vi "ActionVIOnCompile.vi"(8 "error in (no error)":errorcluster, 11 "Device Item Ref in":T1 format="%.0x") -> (0 "error out":errorcluster)   [LabVIEW 2020, in "gRPC Data Server System Explorer.lvlib"]
uses:
  gRPC Data Server System Explorer.lvlib
  <vilib>/NI VeriStand/Custom Device API/Custom Device Item Ref.ctl
  Shared/Compiled.Settings.ctl
  <vilib>/NI VeriStand/Custom Device Tools/Custom Device Utility Library/NI VeriStand - Search for Item by Name.vi
  <vilib>/NI VeriStand/Custom Device API/Set Item Property (Variant).vi
  <vilib>/NI VeriStand/Custom Device Tools/Custom Device Utility Library/Custom Device Utility Library.lvlib
  <vilib>/NI VeriStand/Custom Device API/Custom Device API.lvlib
  <vilib>/NI/NIVS Inline Async API/_Data Access System Explorer/Data Access System Explorer.lvlib
  Shared/gRPC Data Server Shared.lvlib
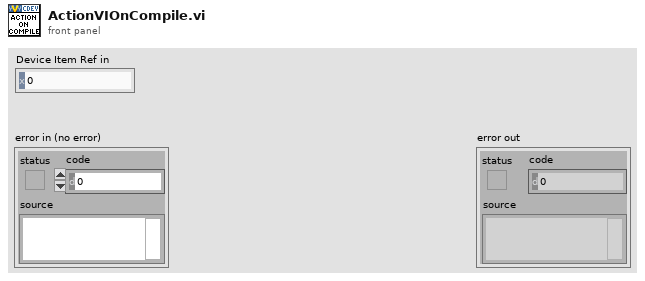
[diagram p1: front panel]
types:
  T1 = typedef "Custom Device API.lvlib/Custom Device Item Ref.ctl" = u64
  T2 = cluster{"Name":string, "Type":enum16{"Output/Write", "Input/Read", "Input/ReadWrite"}, "VS Refs":T1[]}
  T3 = enum16{"Output/Write", "Input/Read", "Input/ReadWrite"}
  T4 = typedef "gRPC Data Server Shared.lvlib/Compiled.Settings.ctl" = cluster{"Name":string, "Server Address":string, "Async?":bool, "Key File":path, "Cert File":path, "Channel Name":string[], "Initial Value":string[]}
  T5 = typedef "Custom Device API.lvlib/Custom Device Item Info.ctl" = cluster{"Name":string, "Is Channel":bool, "GUID":string, "Is Waveform":bool}
  T6 = cluster{"Name":string, "Type":enum16{"Output/Write", "Input/Read", "Input/ReadWrite"}, "VS Refs":T1[]}[]
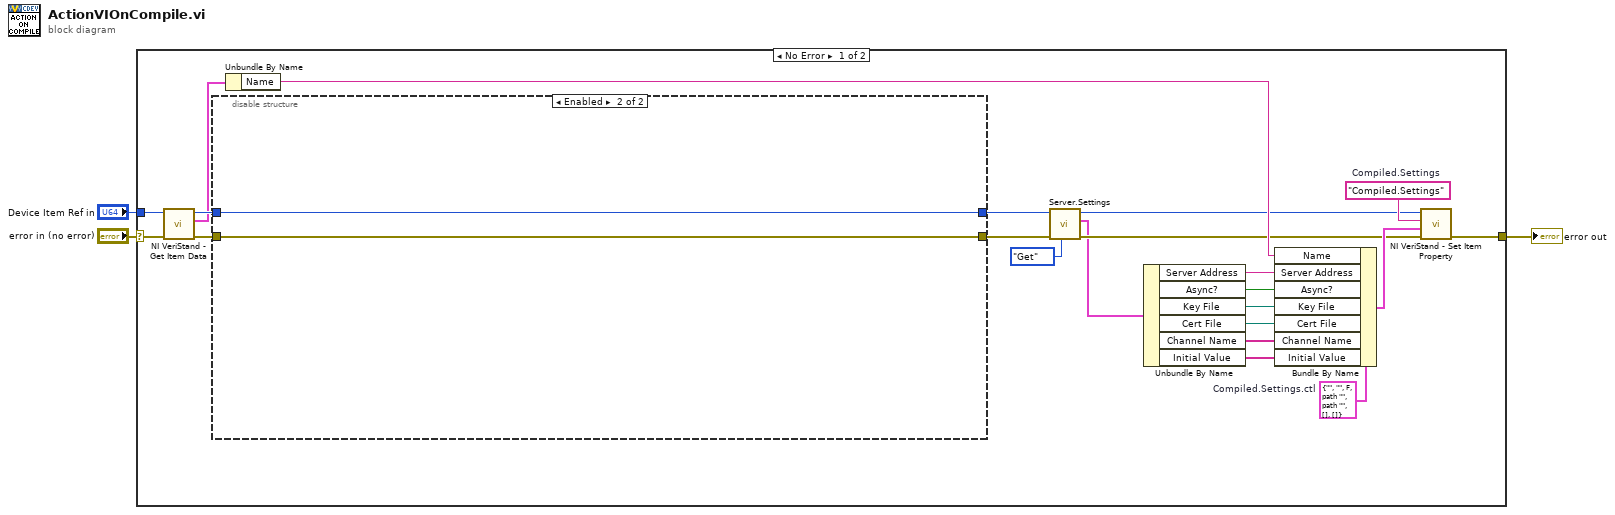
[diagram p0: block diagram]
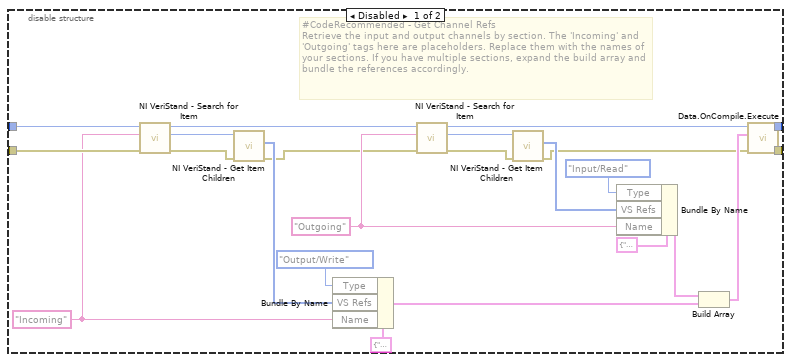
[diagram p2: hidden frame]
diagram:
  n1 = case shown="No Error" "error in (no error)" {
    selector: "error in (no error)" -> [w22 w51]
    tunnel: [w23 w51] -> w2
    tunnel: "Device Item Ref in" -> [w21 _]
    frame No Error {
      w16 = T4 {"Name"="", "Server Address"="", "Async?"=FALSE, "Key File"=path "", "Cert File"=path "", "Channel Name"=[], "Initial Value"=[]}  # Compiled.Settings.ctl
      w25 = "Compiled.Settings"  # Compiled.Settings
      n2 = call <vilib>:"NI VeriStand - Get Item Data.vi"("error in (no error)"=w22, "Item Ref in"=w21) -> ("error out"=w19:errorcluster, "Item Info"=w18:T5, "Item Ref out"=w20:T1)  [unwired: 6 in, 1 out]
      n3 = disable-structure shown="Enabled" {
        disable-tunnel: w20 -> [w44 w50]
        disable-tunnel: w19 -> [w43 w49]
        disable-tunnel: [w27 w49] -> w14
        disable-tunnel: [w26 w50] -> w15
        frame Disabled {
          w40 = "Outgoing" ("Item Name")
          w42 = "Incoming" ("Item Name")
          # "#CodeRecommended - Get Channel Refs\nRetrieve the input and output channels by section. The 'Incoming' and 'Outgoing' tags here are placeholders. Replace them with the names of your sections. If you have multiple sections, expand the build array and bundle the references accordingly."
          n4 = call-poly <vilib>:"NI VeriStand - Search for Item.vi"("error in"=w43, "Item Name"=w42, "Section Ref in"=w44) -> ("error out"=w48:errorcluster, "Item Ref"=w47:T1, "Section Ref out"=w29:T1)  [unwired: 5 in, 1 out]
          n5 = call <vilib>:"NI VeriStand - Get Item Children.vi"("error in (no error)"=w48, "Item Ref in"=w47) -> ("error out"=w28:errorcluster, "Child Refs"=w41:T1[])  [unwired: 6 in, 2 out]
          n6 = Bundle By Name(cluster=T2 {"Name"="", "Type"=enum."Output/Write", "VS Refs"=[]} ("Group"), "Type"=T3."Output/Write", "VS Refs"=w41, "Name"=w42) -> (w32:T2)
          n7 = call-poly <vilib>:"NI VeriStand - Search for Item.vi"("error in"=w28, "Item Name"=w40, "Section Ref in"=w29) -> ("error out"=w45:errorcluster, "Item Ref"=w46:T1, "Section Ref out"=w30:T1)  [unwired: 5 in, 1 out]
          n8 = call <vilib>:"NI VeriStand - Get Item Children.vi"("error in (no error)"=w45, "Item Ref in"=w46) -> ("error out"=w31:errorcluster, "Child Refs"=w36:T1[])  [unwired: 6 in, 2 out]
          n9 = Bundle By Name(cluster=T2 {"Name"="", "Type"=enum."Output/Write", "VS Refs"=[]} ("Group"), "Type"=T3."Input/Read", "VS Refs"=w36, "Name"=w40) -> (w38:T2)
          n10 = Build Array(w38, w32) -> (w35:T6)
          n11 = call <vilib>:"Data.OnCompile.Execute.vi"("error in"=w31, "VS Ref Groups"=w35, "Custom Device Ref"=w30) -> ("error out"=w27:errorcluster, "Custom Device Ref"=w26:T1)  [unwired: 7 in]
        }
        frame Enabled {
        }
      }
      n12 = Unbundle By Name(w18) -> ("Name"=w17:string)
      n13 = call "Server.Settings.vi"("Action"=enum8{"Get", "Set"}."Get", "error in (no error)"=w14, "Parent Ref in"=w15) -> ("error out"=w12:errorcluster, "Client Settings Out"=w10:T4, "Item Ref out"=w13:T1)  [unwired: 6 in]
      n14 = Unbundle By Name(w10) -> ("Server Address"=w9:string, "Async?"=w8:bool, "Key File"=w7:path, "Cert File"=w6:path, "Channel Name"=w5:string[], "Initial Value"=w4:string[])
      n15 = Bundle By Name(cluster=w16, "Name"=w17, "Server Address"=w9, "Async?"=w8, "Key File"=w7, "Cert File"=w6, "Channel Name"=w5, "Initial Value"=w4) -> (w24:T4)
      n16 = call-poly <vilib>:"NI VeriStand - Set Item Property.vi"("error in (no error)"=w12, "Value"=w24, "Property Name"=w25, "Item Ref in"=w13) -> ("error out"=w23:errorcluster)  [unwired: 5 in, 2 out]
    }
    frame Error {
    }
  }
  "error out" <- w2
